vi "matlabwffromparam.vi"(1 "Cluster":T1) -> (0 "Waveform":waveform(dbl))   [LabVIEW 2015]
uses:
  <vilib>/Utility/file.llb/Read Delimited Spreadsheet (DBL).vi
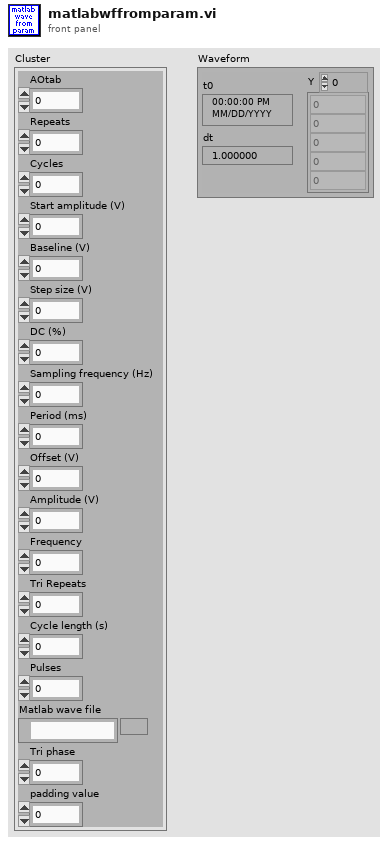
[diagram p1: front panel]
types:
  T1 = cluster{"AOtab":dbl, "Repeats":dbl, "Cycles":dbl, "Start amplitude (V)":dbl, "Baseline (V)":dbl, "Step size (V)":dbl, "DC (%)":dbl, "Sampling frequency (Hz)":dbl, "Period (ms)":dbl, "Offset (V)":dbl, "Amplitude (V)":dbl, "Frequency":dbl, "Tri Repeats":dbl, "Cycle length (s)":dbl, "Pulses":dbl, "Matlab wave file":path, "Tri phase":dbl, "padding value":dbl}
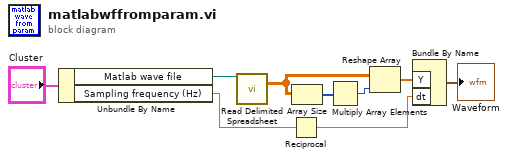
[diagram p0: block diagram]
diagram:
  n1 = Unbundle By Name("Cluster") -> ("Matlab wave file"=w8:path, "Sampling frequency (Hz)"=w9:dbl)
  n2 = call-poly <vilib>:"Read Delimited Spreadsheet.vi"("file path (dialog if empty)"=w8) -> ("all rows"=w5:dbl[][])  [unwired: 9 in, 5 out]
  n3 = Reciprocal(x=w9) -> (1/x=w1:dbl)
  n4 = Array Size(array=w5) -> (size(s)=w4:i32[])
  n5 = Multiply Array Elements(1:w4) -> (0:w3:i32)
  n6 = Reshape Array(w5, w3) -> (w2:dbl[])
  n7 = Bundle By Name("Y"=w2, "dt"=w1) -> (→"Waveform":waveform(dbl))  [unwired: 1 in]
